vi "Alarm Format Hi Lo Cluster.vi"(1 "HI Alarm":T1, 2 "LO Alarm":T1) -> (0 "Limits":cluster{"Lo":dbl, "Hi":dbl}[](array[cluster]))   [LabVIEW 2018]
uses:
  Controls/Alarm Limits TDef.ctl
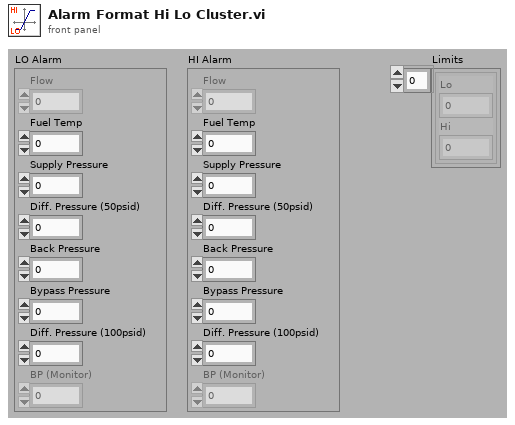
[diagram p1: front panel]
types:
  T1 = typedef "Alarm Limits TDef.ctl" = cluster{"Flow":dbl, "Fuel Temp":dbl, "Supply Pressure":dbl, "Diff. Pressure (50psid)":dbl, "Back Pressure":dbl, "Bypass Pressure":dbl, "Diff. Pressure (100psid)":dbl, "BP (Monitor)":dbl}
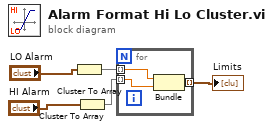
[diagram p0: block diagram]
diagram:
  n1 = Cluster To Array(cluster="LO Alarm") -> (array=w3:dbl[])
  n2 = Cluster To Array(cluster="HI Alarm") -> (array=w2:dbl[])
  n3 = for {
    tunnel: w3 -> [w7] mode=indexing
    tunnel: w2 -> [w6] mode=indexing
    tunnel: [w8] -> w1 mode=indexing
    n4 = Bundle("Flow"=w7, "Flow"=w6) -> (w8:cluster{"Flow":dbl, "Flow":dbl})  [unwired: 1 in]
  }
  "Limits" <- w1
